vi "Close Collection.vi"(8 "error in (no error)":errorcluster, 11 "VI Collection in":refnum<class "VI Collection.lvclass">) -> (0 "error out":errorcluster, 3 "VI Collection out":refnum<class "VI Collection.lvclass">)   [LabVIEW 2013, in "QuickVIew.lvlib" / "VI Collection.lvclass"]
uses:
  VI Collection.lvclass
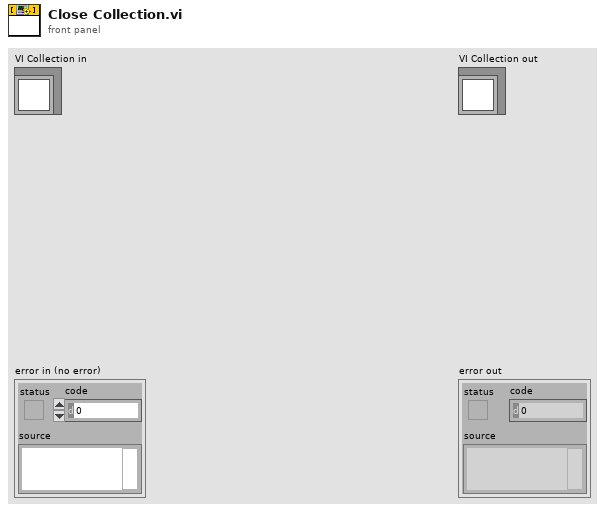
[diagram p1: front panel]
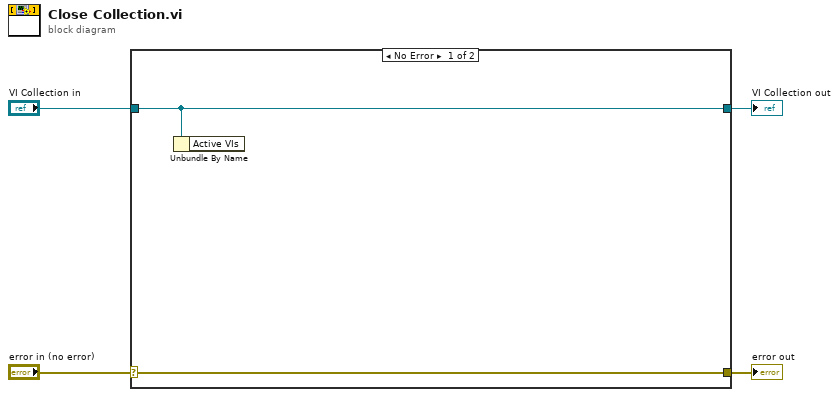
[diagram p0: block diagram]
diagram:
  n1 = case shown="No Error" "error in (no error)" {
    selector: "error in (no error)" -> [w6 w8]
    tunnel: [w6 w8] -> w3
    tunnel: [w5 w7] -> w1
    tunnel: "VI Collection in" -> [w5 w7]
    frame No Error {
      n2 = Unbundle By Name(w5) -> ()  [unwired: 1 out]
    }
    frame Error {
    }
  }
  "error out" <- w3
  "VI Collection out" <- w1
